vi "Check Underflow Error.vi"(2 "error in (no error)":errorcluster, 3 "Underflow Indicator Ref":refnum<vi>, 4 "Filter?":bool) -> (0 "error out":errorcluster, 1 "Underflow?":bool)   [LabVIEW 2020]
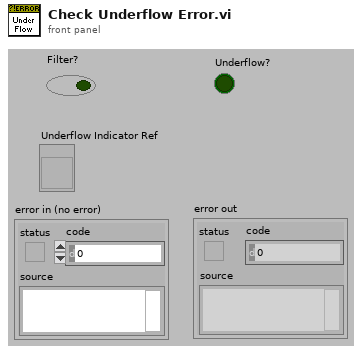
[diagram p1: front panel]
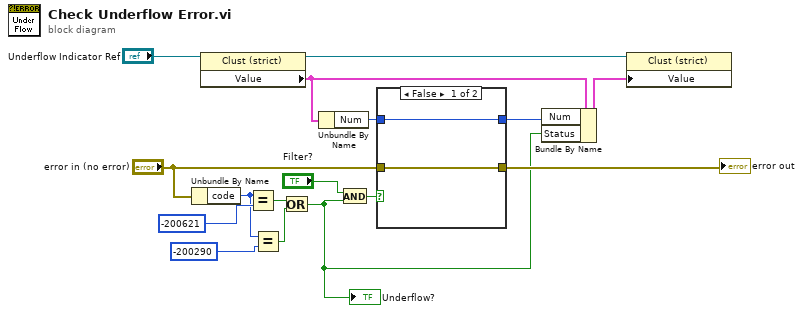
[diagram p0: block diagram]
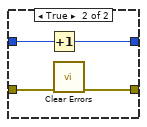
[diagram p2: hidden frame]
diagram:
  n1 = Unbundle By Name("error in (no error)") -> ("code"=w3:i32)
  n2 = property class="Clust (strict)"(reference="Underflow Indicator Ref") -> (reference out=w6:refnum<vi>, "Value"=w8:cluster{"Status":bool, "Num":i32})  [unwired: 1 in, 1 out]
  n3 = Equal?(x=w3, y=-200621 ("code to ignore")) -> (x = y?=w7:bool)
  n4 = Equal?(x=w3, y=-200290 ("code to ignore")) -> (x = y?=w1:bool)
  n5 = Or(x=w7, y=w1) -> (x .or. y?=w4:bool)
  "Underflow?" <- w4
  n6 = Unbundle By Name(w8) -> ("Num"=w10:i32)
  n7 = And(x="Filter?", y=w4) -> (x .and. y?=w13:bool)
  n8 = case shown="False" w13 {
    tunnel: "error in (no error)" -> [w18 w22]
    tunnel: [w18 w21] -> w14
    tunnel: w10 -> [w17 w20]
    tunnel: [w17 w19] -> w9
    frame False {
    }
    frame True {
      n9 = Increment(x=w20) -> (x+1=w19:i32)
      n10 = call <vilib>:"Clear Errors.vi"("error in (no error)"=w22) -> ("error out"=w21:errorcluster)  [unwired: 5 in, 1 out]
    }
  }
  "error out" <- w14
  n11 = Bundle By Name(cluster=w8, "Num"=w9, "Status"=w4) -> (w5:cluster{"Status":bool, "Num":i32})
  n12 = property class="Clust (strict)"(reference=w6, "Value"=w5) -> ()  [unwired: 1 in, 2 out]
